vi "Event Builder.vi"() -> ()   [LabVIEW 2021]
uses:
  CamState.ctl
  <userlib>/FTools/JSON Pretty Printer/JSON Pretty Printer.lvlib
  <vilib>/DAQmx/create/channels.llb/DAQmx Create Channel (DO-Digital Output).vi
  <vilib>/DAQmx/write.llb/DAQmx Write (Digital Bool 1Line 1Point).vi
  <vilib>/DAQmx/create/channels.llb/DAQmx Create Channel (DI-Digital Input).vi
  <vilib>/Field R&D Services/LIBSSH2 for LabVIEW/Toolkit/Channel/Channel.lvclass
  <vilib>/DAQmx/write.llb/DAQmx Write (Digital 1D Bool 1Chan 1Samp).vi
  <vilib>/DAQmx/read.llb/DAQmx Read (Digital 1D Bool 1Chan 1Samp).vi
  <vilib>/DAQmx/read.llb/DAQmx Read (Digital Bool 1Line 1Point).vi
  CamConfig.ctl
panel:
  in  "Preview Cam":enum32{"cam0.local", "cam1.local", "cam2.local"}(radio)
  in  "Preview":bool
  out "cam ip":string[](array[string])=["cam0.local", "cam2.local"]
  out "Enum":T1
  in  "Tab Control":enum32{"Log", "Configuration"}(tab)
  in  "Show Latest":bool
  out "text":string
  in  "Camera Configuration":T2
  in  "Save Config":bool
  out "trig latch":tag="Dev1/port2/line1"
  out "state":tag="Dev1/port2/line5, Dev1/port1/line5, Dev1/port1/line0"
  out "trig reset":tag="Dev1/port2/line0"
  out "trig":tag="Dev1/port2/line1"
  out "enable":tag="Dev1/port2/line5, Dev1/port1/line5, Dev1/port1/line0"
  out "state_com":tag="Dev1/port2/line5, Dev1/port1/line5, Dev1/port1/line0"
  out "Trig Enabled":bool caption="Time has Elapsed"
  in  "Timer Reset":bool
  out "Camera Status":u32[](array[colorbox])
  in  "Start Event":bool
  in  "Manual Trigger":bool
  in  "Capture Frane":bool
  in  "Quit":bool
  out "Event":u32
  out "Time Elapsed (s)":dbl format="%.3f"
  out "Run":string
  out "Triggered":bool
  out "Path":string="C:\\Users\\SBC\\Documents\\Camera_Data\\"
  out "config_path":path=path "C:/Users/SBC/Documents/SBC-EventBuilder/camera_config.json"
  # "Cam 0"
  # "Cam 1"
  # "Cam 2"
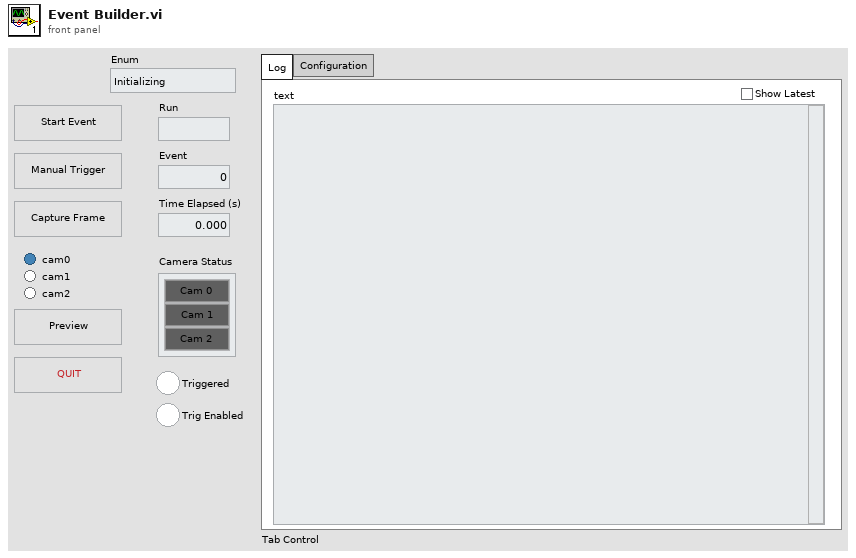
[diagram p1: front panel]
types:
  T1 = typedef "CamState.ctl" = enum16{"Initializing", "Idle", "Starting Event", "Starting RPi", "During Event", "Reset", "Reset RPi", "Preview", "Quit"}
  T2 = typedef "CamConfig.ctl" = cluster{"exposure":u32, "resolution":u32[], "frame_sync":bool, "mode":u32, "buffer_len":u32, "frames_after":u32, "adc_threshold":u32, "pix_threshold":u32, "save_path":string, "config_path":string, "cam_name":string, "image_format":string, "date_format":string, "input_pins":cluster{"state_com":u8, "trig_en":u8, "trig_latch":u8}, "output_pins":cluster{"state":u8, "trig":u8}}
  T3 = enum8{"Enabled", "Disabled", "Disabled and Grayed Out"}
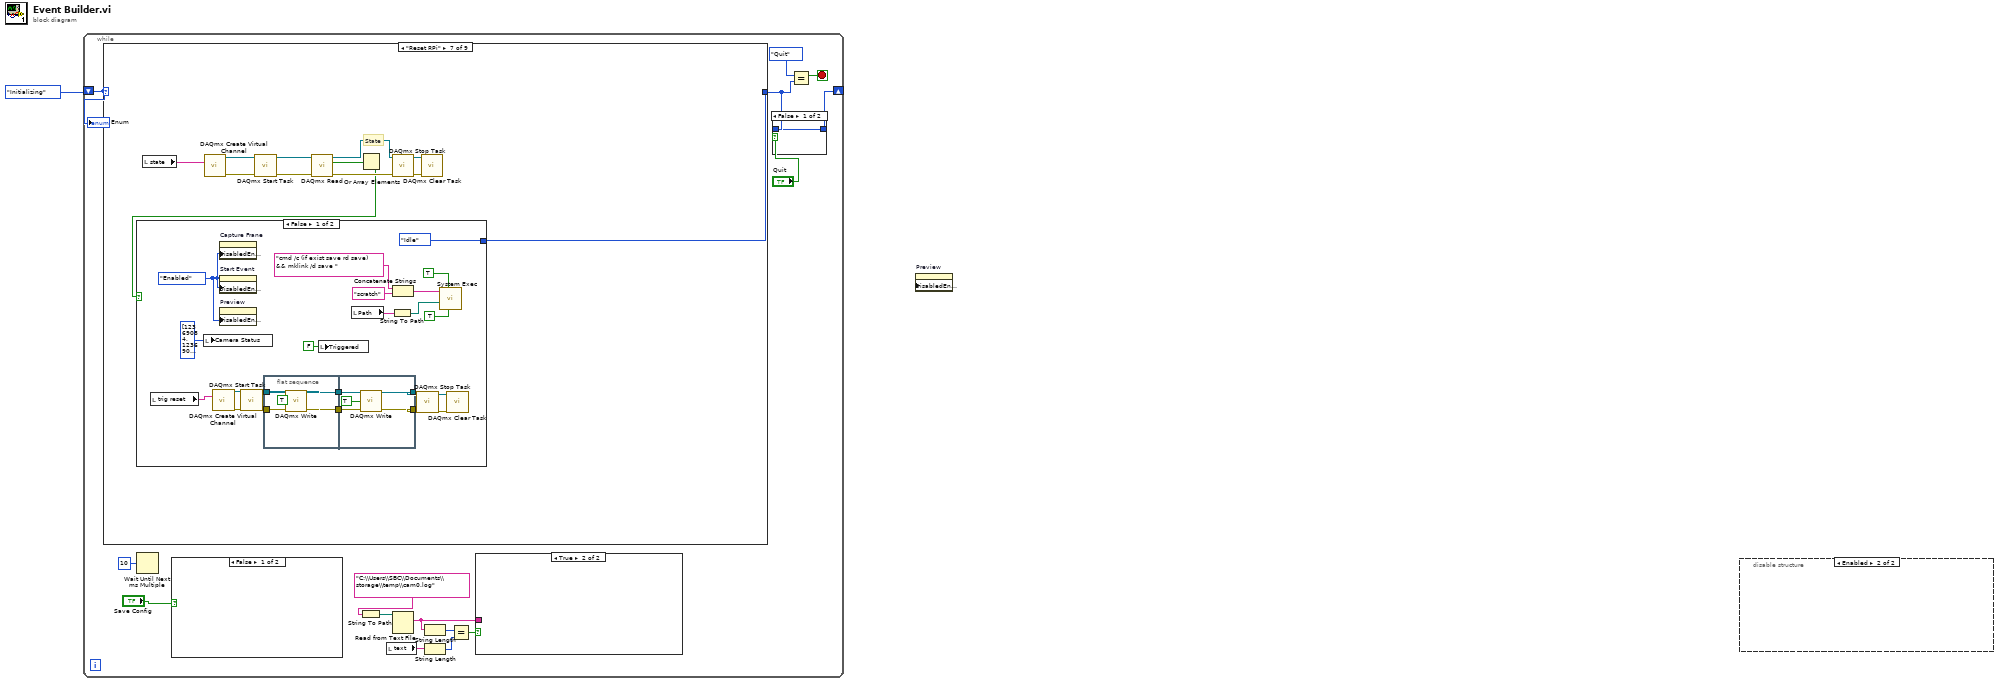
[diagram p0: block diagram]
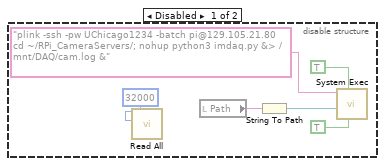
[diagram p2: hidden frame]
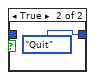
[diagram p3: hidden frame]
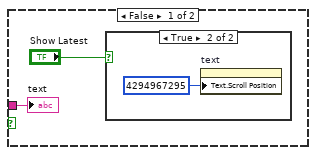
[diagram p4: hidden frame]
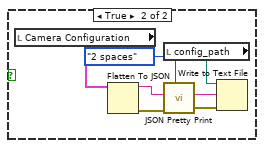
[diagram p6: hidden frame]
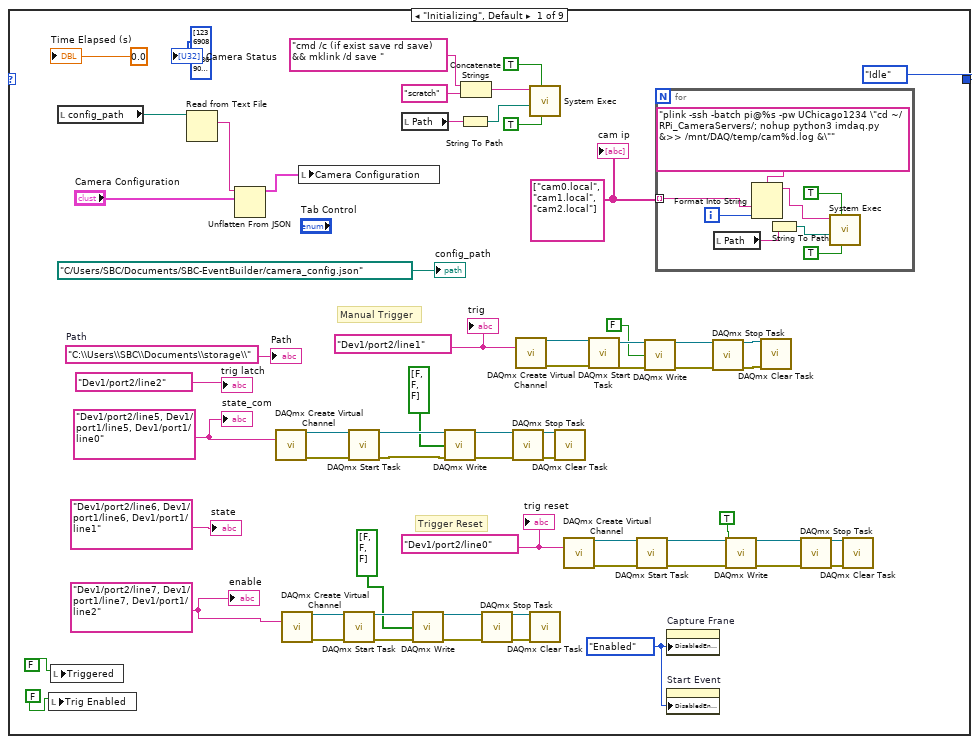
[diagram p7: hidden frame]
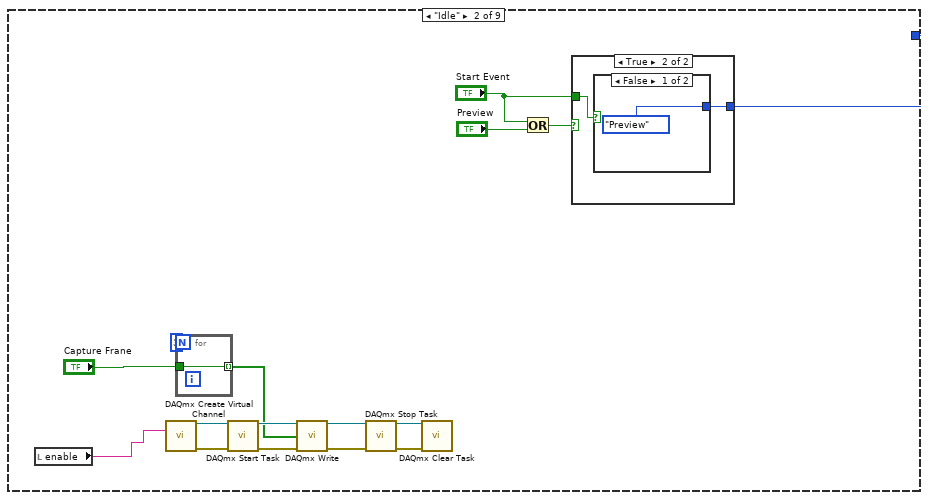
[diagram p8: hidden frame]
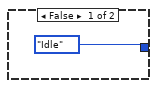
[diagram p9: hidden frame]
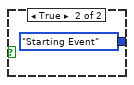
[diagram p10: hidden frame]
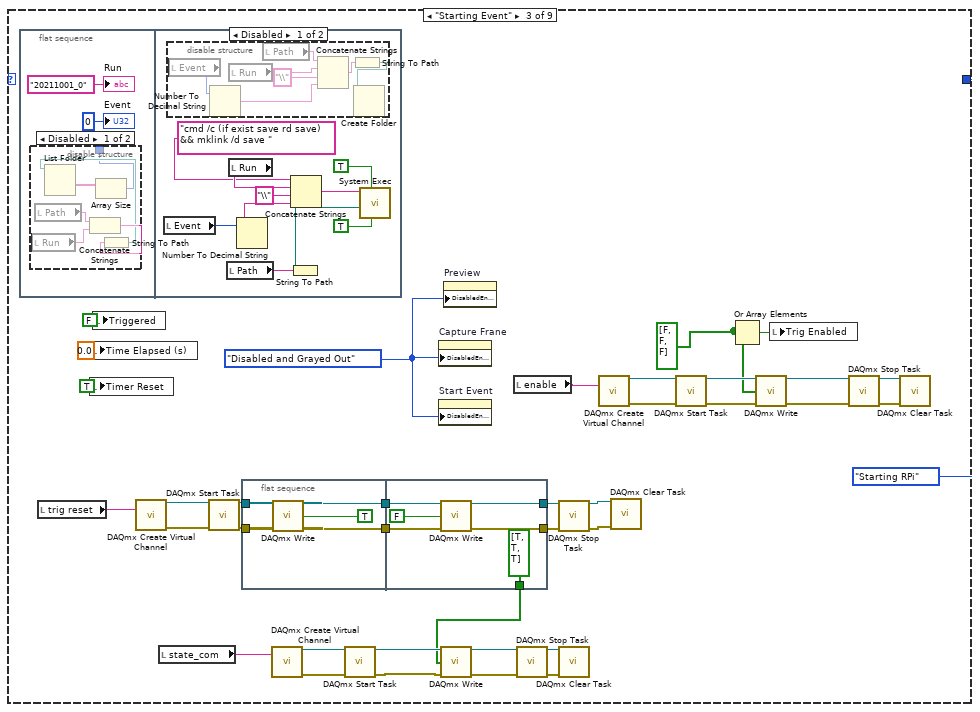
[diagram p11: hidden frame]
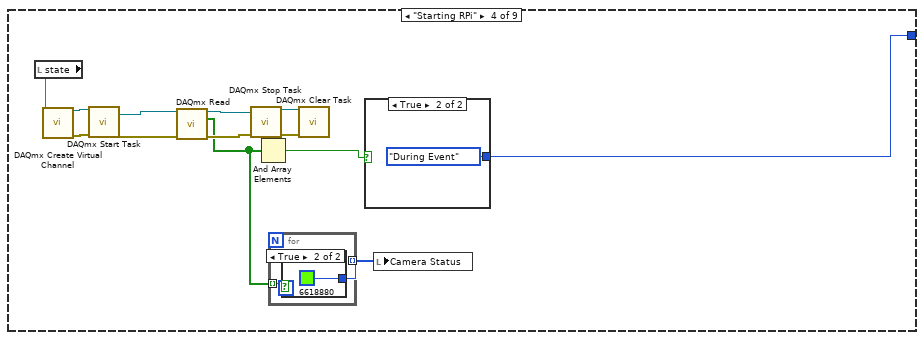
[diagram p14: hidden frame]
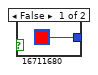
[diagram p15: hidden frame]
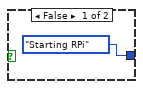
[diagram p16: hidden frame]
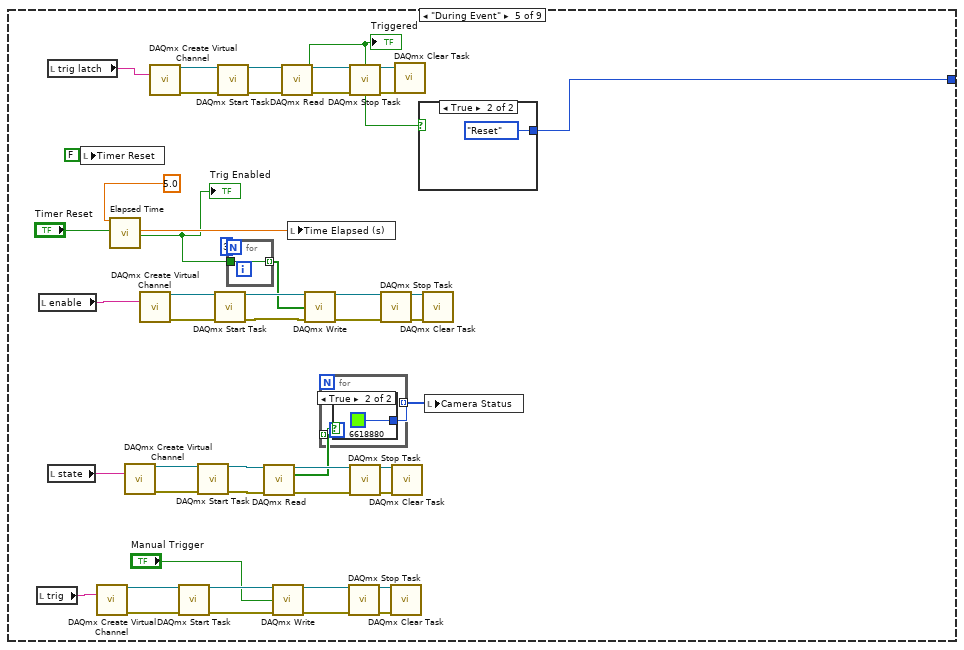
[diagram p17: hidden frame]
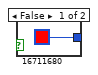
[diagram p18: hidden frame]
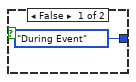
[diagram p19: hidden frame]
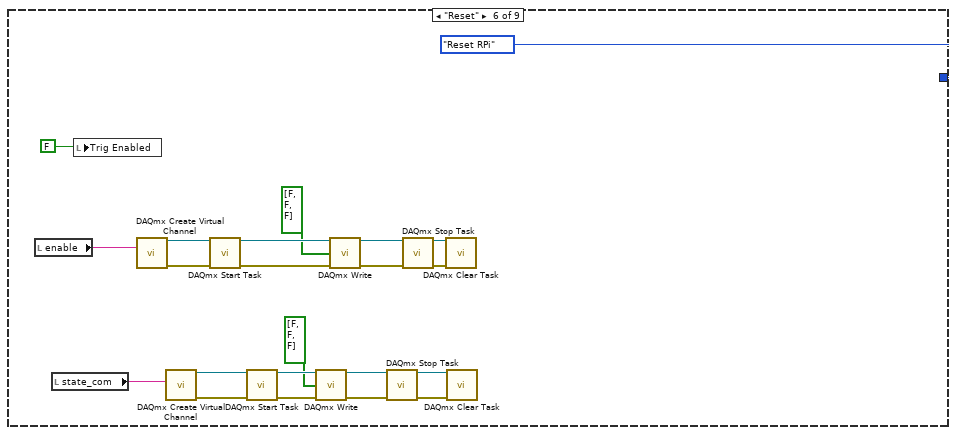
[diagram p20: hidden frame]
diagram:
  n1 = while {
    shift-right: [w5] -> _
    shift-left: CamState."Initializing" -> [w16]
    stop <- w2 stop-if-true
    n2 = case shown="\"Reset RPi\"" w16 {
      tunnel: [CamState."Idle" w114 CamState."Starting RPi" w196 w260 CamState."Reset RPi" w290 CamState."Idle" w365] -> w3
      frame "Initializing", Default {
        w29 = string[] ["cam0.local", "cam1.local", "cam2.local"]
        w32 = tag "Dev1/port2/line7, Dev1/port1/line7, Dev1/port1/line2" ("lines")
        w35 = tag "Dev1/port2/line5, Dev1/port1/line5, Dev1/port1/line0" ("lines")
        w43 = tag "Dev1/port2/line0" ("lines")
        w63 = T3."Enabled" ("Disabled")
        w69 = tag "Dev1/port2/line1" ("lines")
        w62 = "C:\\Users\\SBC\\Documents\\storage\\"  # Path
        # "Trigger Reset"
        # "Manual Trigger"
        n3 = local write "Trig Enabled"(FALSE ("Trig Enabled")) -> ()
        n4 = local write "Triggered"(FALSE ("Triggered")) -> ()
        n5 = local read "config_path"() -> (w86:path)
        n6 = Read from Text File(file (use dialog)=w86) -> (text=w85:string)  [unwired: 3 in, 3 out]
        n7 = Unflatten From JSON(JSON string=w85, type and defaults="Camera Configuration") -> (value=w83:T2)  [unwired: 5 in, 1 out]
        n8 = call-poly <vilib>:"DAQmx Create Virtual Channel.vi"("lines"=w35) -> ("task out"=w53:refnum<k21>, "error out"=w52:errorcluster)  [unwired: 13 in]
        n9 = call-poly <vilib>:"DAQmx Create Virtual Channel.vi"("lines"=w32) -> ("task out"=w79:refnum<k21>, "error out"=w78:errorcluster)  [unwired: 13 in]
        n10 = local write "Camera Configuration"(w83) -> ()
        n11 = call <vilib>:"DAQmx Start Task.vi"("task/channels in"=w79, "error in"=w78) -> ("task out"=w77:refnum<k21>, "error out"=w76:errorcluster)  [unwired: 12 in]
        n12 = call <vilib>:"DAQmx Start Task.vi"("task/channels in"=w53, "error in"=w52) -> ("task out"=w51:refnum<k21>, "error out"=w50:errorcluster)  [unwired: 12 in]
        n13 = local read "Path"() -> (w60:string)
        n14 = call-poly <vilib>:"DAQmx Write.vi"("task/channels in"=w77, "data"=bool[] [FALSE, FALSE, FALSE], "error in"=w76) -> ("task out"=w75:refnum<k21>, "error out"=w74:errorcluster)  [unwired: 10 in, 1 out]
        n15 = call-poly <vilib>:"DAQmx Write.vi"("task/channels in"=w51, "data"=bool[] [FALSE, FALSE, FALSE], "error in"=w50) -> ("task out"=w49:refnum<k21>, "error out"=w48:errorcluster)  [unwired: 10 in, 1 out]
        n16 = String To Path(string=w60) -> (path=w59:path)
        n17 = Concatenate Strings("cmd /c (if exist save rd save) && mklink /d save " ("string"), "scratch" ("string")) -> (w61:string)
        n18 = call <vilib>:"DAQmx Stop Task.vi"("task/channels in"=w75, "error in"=w74) -> ("task out"=w81:refnum<k21>, "error out"=w80:errorcluster)  [unwired: 12 in]
        n19 = call <vilib>:"DAQmx Stop Task.vi"("task/channels in"=w49, "error in"=w48) -> ("task out"=w55:refnum<k21>, "error out"=w54:errorcluster)  [unwired: 12 in]
        n20 = call-poly <vilib>:"DAQmx Create Virtual Channel.vi"("lines"=w69) -> ("task out"=w71:refnum<k21>, "error out"=w70:errorcluster)  [unwired: 13 in]
        n21 = call <vilib>:"System Exec.vi"("run minimized? (F)"=TRUE, "wait until completion? (T)"=TRUE, "working directory"=w59, "command line"=w61) -> ()  [unwired: 4 in, 4 out]
        n22 = call <vilib>:"DAQmx Clear Task.vi"("task in"=w81, "error in"=w80) -> ()  [unwired: 13 in, 1 out]
        n23 = call <vilib>:"DAQmx Clear Task.vi"("task in"=w55, "error in"=w54) -> ()  [unwired: 13 in, 1 out]
        n24 = call-poly <vilib>:"DAQmx Create Virtual Channel.vi"("lines"=w43) -> ("task out"=w45:refnum<k21>, "error out"=w44:errorcluster)  [unwired: 13 in]
        n25 = call <vilib>:"DAQmx Start Task.vi"("task/channels in"=w71, "error in"=w70) -> ("task out"=w68:refnum<k21>, "error out"=w67:errorcluster)  [unwired: 12 in]
        n26 = call <vilib>:"DAQmx Start Task.vi"("task/channels in"=w45, "error in"=w44) -> ("task out"=w41:refnum<k21>, "error out"=w40:errorcluster)  [unwired: 12 in]
        n27 = call-poly <vilib>:"DAQmx Write.vi"("task/channels in"=w68, "data"=FALSE, "error in"=w67) -> ("task out"=w65:refnum<k21>, "error out"=w66:errorcluster)  [unwired: 10 in, 1 out]
        n28 = for {
          tunnel: w29 -> [w92] mode=indexing
          i -> [w91]
          n29 = local read "Path"() -> (w98:string)
          n30 = Format Into String(format string="plink -ssh -batch pi@%s -pw UChicago1234 \"cd ~/RPi_CameraServers/; nohup python3 imdaq.py &>> /mnt/DAQ/temp/cam%d.log &\"" ("string"), w92, w91) -> (resulting string=w93:string)  [unwired: 2 in, 1 out]
          n31 = String To Path(string=w98) -> (path=w97:path)
          n32 = call <vilib>:"System Exec.vi"("run minimized? (F)"=TRUE, "wait until completion? (T)"=TRUE, "working directory"=w97, "command line"=w93) -> ()  [unwired: 4 in, 4 out]
        }
        n33 = property on="Capture Frane" class="Bool"("DisabledEnum"=w63) -> ()  [unwired: 2 in, 2 out]
        n34 = property on="Start Event" class="Bool"("DisabledEnum"=w63) -> ()  [unwired: 2 in, 2 out]
        n35 = call <vilib>:"DAQmx Stop Task.vi"("task/channels in"=w65, "error in"=w66) -> ("task out"=w73:refnum<k21>, "error out"=w72:errorcluster)  [unwired: 12 in]
        n36 = call-poly <vilib>:"DAQmx Write.vi"("task/channels in"=w41, "data"=TRUE, "error in"=w40) -> ("task out"=w39:refnum<k21>, "error out"=w38:errorcluster)  [unwired: 10 in, 1 out]
        n37 = call <vilib>:"DAQmx Clear Task.vi"("task in"=w73, "error in"=w72) -> ()  [unwired: 13 in, 1 out]
        n38 = call <vilib>:"DAQmx Stop Task.vi"("task/channels in"=w39, "error in"=w38) -> ("task out"=w47:refnum<k21>, "error out"=w46:errorcluster)  [unwired: 12 in]
        n39 = call <vilib>:"DAQmx Clear Task.vi"("task in"=w47, "error in"=w46) -> ()  [unwired: 13 in, 1 out]
        "Time Elapsed (s)" <- 0.0 ("Time Elapsed")
        "Camera Status" <- u32[] [12369084, 12369084, 12369084] ("Array")
        "config_path" <- path "C:/Users/SBC/Documents/SBC-EventBuilder/camera_config.json" ("file (use dialog)")
        "Path" <- w62
        "state_com" <- w35
        "enable" <- w32
        "trig" <- w69
        "trig reset" <- w43
        "state" <- tag "Dev1/port2/line6, Dev1/port1/line6, Dev1/port1/line1" ("lines")
        "trig latch" <- tag "Dev1/port2/line2" ("lines")
        "cam ip" <- w29
      }
      frame "Idle" {
        n40 = local read "enable"() -> (w113:tag)
        n41 = call-poly <vilib>:"DAQmx Create Virtual Channel.vi"("lines"=w113) -> ("task out"=w110:refnum<k21>, "error out"=w109:errorcluster)  [unwired: 13 in]
        n42 = for {
          N: 3 -> [_]
          tunnel: [w115] -> w102 mode=indexing
          tunnel: "Capture Frane" -> [w115]
        }
        n43 = call <vilib>:"DAQmx Start Task.vi"("task/channels in"=w110, "error in"=w109) -> ("task out"=w108:refnum<k21>, "error out"=w107:errorcluster)  [unwired: 12 in]
        n44 = call-poly <vilib>:"DAQmx Write.vi"("task/channels in"=w108, "data"=w102, "error in"=w107) -> ("task out"=w106:refnum<k21>, "error out"=w105:errorcluster)  [unwired: 10 in, 1 out]
        n45 = call <vilib>:"DAQmx Stop Task.vi"("task/channels in"=w106, "error in"=w105) -> ("task out"=w112:refnum<k21>, "error out"=w111:errorcluster)  [unwired: 12 in]
        n46 = call <vilib>:"DAQmx Clear Task.vi"("task in"=w112, "error in"=w111) -> ()  [unwired: 13 in, 1 out]
        n47 = Or(x="Start Event", y="Preview") -> (x .or. y?=w100:bool)
        n48 = case shown="True" w100 {
          tunnel: [CamState."Idle" w118] -> w114
          tunnel: "Start Event" -> [_ w117]
          frame False {
          }
          frame True {
            n49 = case shown="False" w117 {
              tunnel: [CamState."Preview" CamState."Starting Event"] -> w118
              frame False {
              }
              frame True {
              }
            }
          }
        }
      }
      frame "Starting Event" {
        w134 = bool[] [FALSE, FALSE, FALSE] ("data")
        w121 = T3."Disabled and Grayed Out" ("Disabled")
        n50 = flat-sequence {
          frame #0 {
            n51 = disable-structure shown="Disabled" {
              disable-tunnel: [w171 _] -> _
              frame Disabled {
                n52 = local read "Run"() -> (w175:string)
                n53 = local read "Path"() -> (w174:string)
                n54 = Concatenate Strings(w174, w175) -> (w173:string)
                n55 = String To Path(string=w173) -> (path=w172:path)
                n56 = List Folder(path=w172) -> (folder names=w176:string[])  [unwired: 3 in, 3 out]
                n57 = Array Size(array=w176) -> (size(s)=w171:i32)
              }
              frame Enabled {
              }
            }
            "Event" <- u32 0 ("Event")
            "Run" <- "20211001_0" ("Run")
          }
          frame #1 {
            n58 = local read "Event"() -> (w181:u32)
            n59 = disable-structure shown="Disabled" {
              frame Disabled {
                n60 = local read "Event"() -> (w188:u32)
                n61 = Number To Decimal String(number=w188) -> (decimal integer string=w187:string)  [unwired: 1 in]
                n62 = local read "Run"() -> (w192:string)
                n63 = local read "Path"() -> (w193:string)
                n64 = Concatenate Strings(w193, w192, "\\" ("string"), w187) -> (w191:string)
                n65 = String To Path(string=w191) -> (path=w190:path)
                n66 = Create Folder(path (use dialog)=w190) -> ()  [unwired: 2 in, 3 out]
              }
              frame Enabled {
              }
            }
            n67 = local read "Path"() -> (w184:string)
            n68 = local read "Run"() -> (w182:string)
            n69 = Number To Decimal String(number=w181) -> (decimal integer string=w180:string)  [unwired: 1 in]
            n70 = String To Path(string=w184) -> (path=w183:path)
            n71 = Concatenate Strings("cmd /c (if exist save rd save) && mklink /d save " ("string"), w182, "\\" ("string"), w180) -> (w186:string)
            n72 = call <vilib>:"System Exec.vi"("run minimized? (F)"=TRUE, "wait until completion? (T)"=TRUE, "working directory"=w183, "command line"=w186) -> ()  [unwired: 4 in, 4 out]
          }
        }
        n73 = local read "trig reset"() -> (w133:tag)
        n74 = local write "Time Elapsed (s)"(0.0 ("Time Elapsed (s)")) -> ()
        n75 = local write "Timer Reset"(TRUE ("Timer Reset")) -> ()
        n76 = local write "Triggered"(FALSE ("Triggered")) -> ()
        n77 = call-poly <vilib>:"DAQmx Create Virtual Channel.vi"("lines"=w133) -> ("task out"=w153:refnum<k21>, "error out"=w152:errorcluster)  [unwired: 13 in]
        n78 = local read "state_com"() -> (w123:tag)
        n79 = call <vilib>:"DAQmx Start Task.vi"("task/channels in"=w153, "error in"=w152) -> ("task out"=w151:refnum<k21>, "error out"=w150:errorcluster)  [unwired: 12 in]
        n80 = flat-sequence {
          tunnel: w151 -> [w162]
          tunnel: w150 -> [w161]
          tunnel: [w159] -> w147
          tunnel: [w158] -> w146
          tunnel: [w168] -> w149
          tunnel: [w167] -> w148
          tunnel: w147 -> [w165]
          tunnel: w146 -> [w164]
          tunnel: [bool[] [TRUE, TRUE, TRUE] ("data")] -> w122
          frame #0 {
            n81 = call-poly <vilib>:"DAQmx Write.vi"("task/channels in"=w162, "data"=TRUE, "error in"=w161) -> ("task out"=w158:refnum<k21>, "error out"=w159:errorcluster)  [unwired: 10 in, 1 out]
          }
          frame #1 {
            n82 = call-poly <vilib>:"DAQmx Write.vi"("task/channels in"=w164, "data"=FALSE, "error in"=w165) -> ("task out"=w168:refnum<k21>, "error out"=w167:errorcluster)  [unwired: 10 in, 1 out]
          }
        }
        n83 = call-poly <vilib>:"DAQmx Create Virtual Channel.vi"("lines"=w123) -> ("task out"=w129:refnum<k21>, "error out"=w128:errorcluster)  [unwired: 13 in]
        n84 = call <vilib>:"DAQmx Start Task.vi"("task/channels in"=w129, "error in"=w128) -> ("task out"=w127:refnum<k21>, "error out"=w126:errorcluster)  [unwired: 12 in]
        n85 = property on="Capture Frane" class="Bool"("DisabledEnum"=w121) -> ()  [unwired: 2 in, 2 out]
        n86 = property on="Start Event" class="Bool"("DisabledEnum"=w121) -> ()  [unwired: 2 in, 2 out]
        n87 = call-poly <vilib>:"DAQmx Write.vi"("task/channels in"=w127, "data"=w122, "error in"=w126) -> ("task out"=w125:refnum<k21>, "error out"=w124:errorcluster)  [unwired: 10 in, 1 out]
        n88 = property on="Preview" class="Bool"("DisabledEnum"=w121) -> ()  [unwired: 2 in, 2 out]
        n89 = local read "enable"() -> (w136:tag)
        n90 = call <vilib>:"DAQmx Stop Task.vi"("task/channels in"=w125, "error in"=w124) -> ("task out"=w131:refnum<k21>, "error out"=w130:errorcluster)  [unwired: 12 in]
        n91 = call <vilib>:"DAQmx Stop Task.vi"("task/channels in"=w149, "error in"=w148) -> ("task out"=w155:refnum<k21>, "error out"=w154:errorcluster)  [unwired: 12 in]
        n92 = call <vilib>:"DAQmx Clear Task.vi"("task in"=w131, "error in"=w130) -> ()  [unwired: 13 in, 1 out]
        n93 = call-poly <vilib>:"DAQmx Create Virtual Channel.vi"("lines"=w136) -> ("task out"=w143:refnum<k21>, "error out"=w142:errorcluster)  [unwired: 13 in]
        n94 = call <vilib>:"DAQmx Clear Task.vi"("task in"=w155, "error in"=w154) -> ()  [unwired: 13 in, 1 out]
        n95 = call <vilib>:"DAQmx Start Task.vi"("task/channels in"=w143, "error in"=w142) -> ("task out"=w141:refnum<k21>, "error out"=w140:errorcluster)  [unwired: 12 in]
        n96 = Or Array Elements(Boolean array=w134) -> (logical OR=w135:bool)
        n97 = call-poly <vilib>:"DAQmx Write.vi"("task/channels in"=w141, "data"=w134, "error in"=w140) -> ("task out"=w139:refnum<k21>, "error out"=w138:errorcluster)  [unwired: 10 in, 1 out]
        n98 = local write "Trig Enabled"(w135) -> ()
        n99 = call <vilib>:"DAQmx Stop Task.vi"("task/channels in"=w139, "error in"=w138) -> ("task out"=w145:refnum<k21>, "error out"=w144:errorcluster)  [unwired: 12 in]
        n100 = call <vilib>:"DAQmx Clear Task.vi"("task in"=w145, "error in"=w144) -> ()  [unwired: 13 in, 1 out]
      }
      frame "Starting RPi" {
        n101 = local read "state"() -> (w200:tag)
        n102 = call-poly <vilib>:"DAQmx Create Virtual Channel.vi"("lines"=w200) -> ("task out"=w199:refnum<k21>, "error out"=w204:errorcluster)  [unwired: 13 in]
        n103 = call <vilib>:"DAQmx Start Task.vi"("task/channels in"=w199, "error in"=w204) -> ("task out"=w198:refnum<k21>, "error out"=w203:errorcluster)  [unwired: 12 in]
        n104 = call-poly <vilib>:"DAQmx Read.vi"("task/channels in"=w198, "error in"=w203) -> ("task out"=w202:refnum<k21>, "data"=w194:bool[], "error out"=w201:errorcluster)  [unwired: 11 in]
        n105 = call <vilib>:"DAQmx Stop Task.vi"("task/channels in"=w202, "error in"=w201) -> ("task out"=w206:refnum<k21>, "error out"=w205:errorcluster)  [unwired: 12 in]
        n106 = And Array Elements(Boolean array=w194) -> (logical AND=w197:bool)
        n107 = for {
          tunnel: [w208] -> w195 mode=indexing
          tunnel: w194 -> [w207] mode=indexing
          n108 = case shown="True" w207 {
            tunnel: [u32 16711680 ("Camera Alive") u32 6618880 ("Camera Alive")] -> w208
            frame False {
            }
            frame True {
            }
          }
        }
        n109 = call <vilib>:"DAQmx Clear Task.vi"("task in"=w206, "error in"=w205) -> ()  [unwired: 13 in, 1 out]
        n110 = case shown="True" w197 {
          tunnel: [CamState."Starting RPi" CamState."During Event"] -> w196
          frame False {
          }
          frame True {
          }
        }
        n111 = local write "Camera Status"(w195) -> ()
      }
      frame "During Event" {
        n112 = local read "trig"() -> (w217:tag)
        n113 = local read "enable"() -> (w220:tag)
        n114 = local read "trig latch"() -> (w218:tag)
        n115 = local read "state"() -> (w219:tag)
        n116 = local write "Timer Reset"(FALSE) -> ()
        n117 = call-poly <vilib>:"DAQmx Create Virtual Channel.vi"("lines"=w217) -> ("task out"=w247:refnum<k21>, "error out"=w246:errorcluster)  [unwired: 13 in]
        n118 = call "Elapsed Time"("Time Target (s)"=5.0, "Reset"="Timer Reset") -> ("Elapsed Time (s)"=w259:dbl, "Time has Elapsed"=w215:bool)  [unwired: 10 in, 6 out]
        "Trig Enabled" <- w215
        n119 = call-poly <vilib>:"DAQmx Create Virtual Channel.vi"("lines"=w219) -> ("task out"=w236:refnum<k21>, "error out"=w237:errorcluster)  [unwired: 13 in]
        n120 = call-poly <vilib>:"DAQmx Create Virtual Channel.vi"("lines"=w220) -> ("task out"=w256:refnum<k21>, "error out"=w255:errorcluster)  [unwired: 13 in]
        n121 = call-poly <vilib>:"DAQmx Create Virtual Channel.vi"("lines"=w218) -> ("task out"=w230:refnum<k21>, "error out"=w231:errorcluster)  [unwired: 13 in]
        n122 = call <vilib>:"DAQmx Start Task.vi"("task/channels in"=w247, "error in"=w246) -> ("task out"=w245:refnum<k21>, "error out"=w244:errorcluster)  [unwired: 12 in]
        n123 = call <vilib>:"DAQmx Start Task.vi"("task/channels in"=w236, "error in"=w237) -> ("task out"=w235:refnum<k21>, "error out"=w234:errorcluster)  [unwired: 12 in]
        n124 = call <vilib>:"DAQmx Start Task.vi"("task/channels in"=w256, "error in"=w255) -> ("task out"=w254:refnum<k21>, "error out"=w253:errorcluster)  [unwired: 12 in]
        n125 = call <vilib>:"DAQmx Start Task.vi"("task/channels in"=w230, "error in"=w231) -> ("task out"=w229:refnum<k21>, "error out"=w228:errorcluster)  [unwired: 12 in]
        n126 = for {
          N: 3 -> [_]
          tunnel: w215 -> [w265]
          tunnel: [w265] -> w214 mode=indexing
        }
        n127 = call-poly <vilib>:"DAQmx Read.vi"("task/channels in"=w235, "error in"=w234) -> ("task out"=w233:refnum<k21>, "data"=w216:bool[], "error out"=w232:errorcluster)  [unwired: 11 in]
        n128 = call-poly <vilib>:"DAQmx Write.vi"("task/channels in"=w245, "data"="Manual Trigger", "error in"=w244) -> ("task out"=w241:refnum<k21>, "error out"=w243:errorcluster)  [unwired: 10 in, 1 out]
        n129 = call-poly <vilib>:"DAQmx Read.vi"("task/channels in"=w229, "error in"=w228) -> ("task out"=w227:refnum<k21>, "data"=w225:bool, "error out"=w226:errorcluster)  [unwired: 11 in]
        "Triggered" <- w225
        n130 = local write "Time Elapsed (s)"(w259) -> ()
        n131 = call-poly <vilib>:"DAQmx Write.vi"("task/channels in"=w254, "data"=w214, "error in"=w253) -> ("task out"=w252:refnum<k21>, "error out"=w251:errorcluster)  [unwired: 10 in, 1 out]
        n132 = for {
          tunnel: [w262] -> w250 mode=indexing
          tunnel: w216 -> [w261] mode=indexing
          n133 = case shown="True" w261 {
            tunnel: [u32 16711680 ("Camera Alive") u32 6618880 ("Camera Alive")] -> w262
            frame False {
            }
            frame True {
            }
          }
        }
        n134 = call <vilib>:"DAQmx Stop Task.vi"("task/channels in"=w241, "error in"=w243) -> ("task out"=w249:refnum<k21>, "error out"=w248:errorcluster)  [unwired: 12 in]
        n135 = call <vilib>:"DAQmx Stop Task.vi"("task/channels in"=w227, "error in"=w226) -> ("task out"=w224:refnum<k21>, "error out"=w223:errorcluster)  [unwired: 12 in]
        n136 = call <vilib>:"DAQmx Stop Task.vi"("task/channels in"=w233, "error in"=w232) -> ("task out"=w222:refnum<k21>, "error out"=w221:errorcluster)  [unwired: 12 in]
        n137 = call <vilib>:"DAQmx Stop Task.vi"("task/channels in"=w252, "error in"=w251) -> ("task out"=w258:refnum<k21>, "error out"=w257:errorcluster)  [unwired: 12 in]
        n138 = call <vilib>:"DAQmx Clear Task.vi"("task in"=w249, "error in"=w248) -> ()  [unwired: 13 in, 1 out]
        n139 = call <vilib>:"DAQmx Clear Task.vi"("task in"=w222, "error in"=w221) -> ()  [unwired: 13 in, 1 out]
        n140 = call <vilib>:"DAQmx Clear Task.vi"("task in"=w224, "error in"=w223) -> ()  [unwired: 13 in, 1 out]
        n141 = case shown="True" w225 {
          tunnel: [CamState."During Event" CamState."Reset"] -> w260
          frame False {
          }
          frame True {
          }
        }
        n142 = call <vilib>:"DAQmx Clear Task.vi"("task in"=w258, "error in"=w257) -> ()  [unwired: 13 in, 1 out]
        n143 = local write "Camera Status"(w250) -> ()
      }
      frame "Reset" {
        n144 = local read "enable"() -> (w271:tag)
        n145 = local read "state_com"() -> (w270:tag)
        n146 = local write "Trig Enabled"(FALSE ("Trig Enabled")) -> ()
        n147 = call-poly <vilib>:"DAQmx Create Virtual Channel.vi"("lines"=w271) -> ("task out"=w287:refnum<k21>, "error out"=w286:errorcluster)  [unwired: 13 in]
        n148 = call-poly <vilib>:"DAQmx Create Virtual Channel.vi"("lines"=w270) -> ("task out"=w279:refnum<k21>, "error out"=w278:errorcluster)  [unwired: 13 in]
        n149 = call <vilib>:"DAQmx Start Task.vi"("task/channels in"=w287, "error in"=w286) -> ("task out"=w285:refnum<k21>, "error out"=w284:errorcluster)  [unwired: 12 in]
        n150 = call <vilib>:"DAQmx Start Task.vi"("task/channels in"=w279, "error in"=w278) -> ("task out"=w277:refnum<k21>, "error out"=w276:errorcluster)  [unwired: 12 in]
        n151 = call-poly <vilib>:"DAQmx Write.vi"("task/channels in"=w277, "data"=bool[] [FALSE, FALSE, FALSE], "error in"=w276) -> ("task out"=w275:refnum<k21>, "error out"=w274:errorcluster)  [unwired: 10 in, 1 out]
        n152 = call-poly <vilib>:"DAQmx Write.vi"("task/channels in"=w285, "data"=bool[] [FALSE, FALSE, FALSE], "error in"=w284) -> ("task out"=w283:refnum<k21>, "error out"=w282:errorcluster)  [unwired: 10 in, 1 out]
        n153 = call <vilib>:"DAQmx Stop Task.vi"("task/channels in"=w275, "error in"=w274) -> ("task out"=w281:refnum<k21>, "error out"=w280:errorcluster)  [unwired: 12 in]
        n154 = call <vilib>:"DAQmx Stop Task.vi"("task/channels in"=w283, "error in"=w282) -> ("task out"=w289:refnum<k21>, "error out"=w288:errorcluster)  [unwired: 12 in]
        n155 = call <vilib>:"DAQmx Clear Task.vi"("task in"=w289, "error in"=w288) -> ()  [unwired: 13 in, 1 out]
        n156 = call <vilib>:"DAQmx Clear Task.vi"("task in"=w281, "error in"=w280) -> ()  [unwired: 13 in, 1 out]
      }
      frame "Reset RPi" {
        # "State"
        n157 = local read "state"() -> (w293:tag)
        n158 = call-poly <vilib>:"DAQmx Create Virtual Channel.vi"("lines"=w293) -> ("task out"=w296:refnum<k21>, "error out"=w297:errorcluster)  [unwired: 13 in]
        n159 = call <vilib>:"DAQmx Start Task.vi"("task/channels in"=w296, "error in"=w297) -> ("task out"=w298:refnum<k21>, "error out"=w299:errorcluster)  [unwired: 12 in]
        n160 = call-poly <vilib>:"DAQmx Read.vi"("task/channels in"=w298, "error in"=w299) -> ("task out"=w300:refnum<k21>, "data"=w292:bool[], "error out"=w301:errorcluster)  [unwired: 11 in]
        n161 = Or Array Elements(Boolean array=w292) -> (logical OR=w291:bool)
        n162 = case shown="False" w291 {
          tunnel: [CamState."Idle" CamState."Reset RPi"] -> w290
          frame False {
            w302 = T3."Enabled" ("Disabled")
            n163 = local read "trig reset"() -> (w303:tag)
            n164 = local write "Camera Status"(u32[] [12369084, 12369084, 12369084] ("Array")) -> ()
            n165 = call-poly <vilib>:"DAQmx Create Virtual Channel.vi"("lines"=w303) -> ("task out"=w309:refnum<k21>, "error out"=w308:errorcluster)  [unwired: 13 in]
            n166 = property on="Capture Frane" class="Bool"("DisabledEnum"=w302) -> ()  [unwired: 2 in, 2 out]
            n167 = property on="Start Event" class="Bool"("DisabledEnum"=w302) -> ()  [unwired: 2 in, 2 out]
            n168 = property on="Preview" class="Bool"("DisabledEnum"=w302) -> ()  [unwired: 2 in, 2 out]
            n169 = call <vilib>:"DAQmx Start Task.vi"("task/channels in"=w309, "error in"=w308) -> ("task out"=w307:refnum<k21>, "error out"=w306:errorcluster)  [unwired: 12 in]
            n170 = flat-sequence {
              tunnel: w307 -> [w328]
              tunnel: w306 -> [w327]
              tunnel: [w325] -> w313
              tunnel: [w324] -> w312
              tunnel: [w333] -> w305
              tunnel: [w332] -> w304
              tunnel: w313 -> [w330]
              tunnel: w312 -> [w329]
              frame #0 {
                n171 = call-poly <vilib>:"DAQmx Write.vi"("task/channels in"=w328, "data"=TRUE, "error in"=w327) -> ("task out"=w324:refnum<k21>, "error out"=w325:errorcluster)  [unwired: 10 in, 1 out]
              }
              frame #1 {
                n172 = call-poly <vilib>:"DAQmx Write.vi"("task/channels in"=w329, "data"=TRUE, "error in"=w330) -> ("task out"=w333:refnum<k21>, "error out"=w332:errorcluster)  [unwired: 10 in, 1 out]
              }
            }
            n173 = local write "Triggered"(FALSE ("Triggered")) -> ()
            n174 = local read "Path"() -> (w321:string)
            n175 = String To Path(string=w321) -> (path=w320:path)
            n176 = Concatenate Strings("cmd /c (if exist save rd save) && mklink /d save " ("string"), "scratch" ("string")) -> (w322:string)
            n177 = call <vilib>:"DAQmx Stop Task.vi"("task/channels in"=w305, "error in"=w304) -> ("task out"=w311:refnum<k21>, "error out"=w310:errorcluster)  [unwired: 12 in]
            n178 = call <vilib>:"System Exec.vi"("run minimized? (F)"=TRUE, "wait until completion? (T)"=TRUE, "working directory"=w320, "command line"=w322) -> ()  [unwired: 4 in, 4 out]
            n179 = call <vilib>:"DAQmx Clear Task.vi"("task in"=w311, "error in"=w310) -> ()  [unwired: 13 in, 1 out]
          }
          frame True {
          }
        }
        n180 = call <vilib>:"DAQmx Stop Task.vi"("task/channels in"=w300, "error in"=w301) -> ("task out"=w294:refnum<k21>, "error out"=w295:errorcluster)  [unwired: 12 in]
        n181 = call <vilib>:"DAQmx Clear Task.vi"("task in"=w294, "error in"=w295) -> ()  [unwired: 13 in, 1 out]
      }
      frame "Preview" {
        (unwired) "cmd /c C:\\\\Program^ Files^ ^(x86^)\\\\gstreamer\\\\1.0\\\\mingw_x86_64\\\\bin\\\\gst-launch-1.0 -v tcpclientsrc host=%s port=%d ! decodebin ! autovideosink" ("command line")
        w350 = 5000 ("input 2")
        n182 = local read "Path"() -> (w349:string)
        n183 = Format Into String(format string="plink -ssh -batch pi@%s -pw UChicago1234 \"pkill -f \\\\\\\"imdaq.py\\\\\\\"\"" ("string"), "Preview Cam") -> (resulting string=w347:string)  [unwired: 2 in, 1 out]
        n184 = String To Path(string=w349) -> (path=w348:path)
        n185 = call <vilib>:"System Exec.vi"("run minimized? (F)"=TRUE, "wait until completion? (T)"=TRUE, "working directory"=w348, "command line"=w347) -> ("error out"=w343:errorcluster)  [unwired: 4 in, 3 out]
        n186 = local read "Path"() -> (w361:string)
        n187 = Format Into String(format string="plink -ssh -batch pi@%s -pw UChicago1234 \"~/RPi_CameraServers/MIPI_Camera/RPI/video2stdout | nc -l -p %d\"" ("string"), "Preview Cam", w350) -> (resulting string=w357:string)  [unwired: 2 in, 1 out]
        n188 = String To Path(string=w361) -> (path=w360:path)
        n189 = call <vilib>:"System Exec.vi"("run minimized? (F)"=TRUE, "wait until completion? (T)"=FALSE, "error in (no error)"=w343, "working directory"=w360, "command line"=w357) -> ("error out"=w354:errorcluster)  [unwired: 3 in, 3 out]
        n190 = local read "Path"() -> (w355:string)
        n191 = Format Into String(format string="C:\\\\Program Files (x86)\\\\gstreamer\\\\1.0\\\\mingw_x86_64\\\\bin\\\\gst-launch-1.0 -v tcpclientsrc host=%s port=%d ! decodebin ! autovideosink" ("command line"), "Preview Cam", w350) -> (resulting string=w351:string)  [unwired: 2 in, 1 out]
        n192 = String To Path(string=w355) -> (path=w364:path)
        n193 = call <vilib>:"System Exec.vi"("run minimized? (F)"=TRUE, "wait until completion? (T)"=TRUE, "error in (no error)"=w354, "working directory"=w364, "command line"=w351) -> ()  [unwired: 3 in, 4 out]
        n194 = local read "Path"() -> (w342:string)
        n195 = Format Into String(format string="plink -ssh -batch pi@%s -pw UChicago1234 \"cd ~/RPi_CameraServers/; nohup python3 imdaq.py &>> /mnt/DAQ/temp/cam%d.log &\"" ("string"), "Preview Cam", 0 ("input 2")) -> (resulting string=w340:string)  [unwired: 2 in, 1 out]
        n196 = String To Path(string=w342) -> (path=w341:path)
        n197 = call <vilib>:"System Exec.vi"("run minimized? (F)"=TRUE, "wait until completion? (T)"=TRUE, "working directory"=w341, "command line"=w340) -> ()  [unwired: 4 in, 4 out]
      }
      frame "Quit" {
        n198 = flat-sequence {
          tunnel: [CamState."Quit"] -> w365
          frame #0 {
            w369 = T3."Enabled" ("Disabled")
            n199 = local write "Camera Status"(u32[] [12369084, 12369084, 12369084] ("Array")) -> ()
            n200 = property on="Capture Frane" class="Bool"("DisabledEnum"=w369) -> ()  [unwired: 2 in, 2 out]
            n201 = property on="Start Event" class="Bool"("DisabledEnum"=w369) -> ()  [unwired: 2 in, 2 out]
            n202 = local read "Path"() -> (w375:string)
            n203 = String To Path(string=w375) -> (path=w374:path)
            n204 = Concatenate Strings("cmd /c (if exist save rd save) && mklink /d save " ("string"), "scratch" ("string")) -> (w376:string)
            n205 = local write "Trig Enabled"(FALSE ("Trig Enabled")) -> ()
            n206 = local write "Triggered"(FALSE ("Triggered")) -> ()
            n207 = call <vilib>:"System Exec.vi"("run minimized? (F)"=TRUE, "wait until completion? (T)"=TRUE, "working directory"=w374, "command line"=w376) -> ()  [unwired: 4 in, 4 out]
          }
          frame #1 {
            n208 = local read "cam ip"() -> (w377:string[])
            n209 = for {
              tunnel: w377 -> [w378] mode=indexing
              n210 = local read "Path"() -> (w384:string)
              n211 = Format Into String(format string="plink -ssh -batch pi@%s -pw UChicago1234 \"pkill -f \\\"imdaq.py\\\"\"" ("string"), w378) -> (resulting string=w379:string)  [unwired: 2 in, 1 out]
              n212 = String To Path(string=w384) -> (path=w383:path)
              n213 = call <vilib>:"System Exec.vi"("run minimized? (F)"=TRUE, "wait until completion? (T)"=TRUE, "working directory"=w383, "command line"=w379) -> ()  [unwired: 4 in, 4 out]
            }
          }
          frame #2 {
          }
        }
      }
    }
    n214 = Wait Until Next ms Multiple(millisecond multiple=u32 10) -> ()  [unwired: 1 out]
    n215 = case shown="False" "Save Config" {
      frame False {
      }
      frame True {
        n216 = local read "Camera Configuration"() -> (w28:T2)
        n217 = Flatten To JSON(anything=w28) -> (JSON string=w26:string, 11:w25:errorcluster)  [unwired: 2 in]
        n218 = local read "config_path"() -> (w27:path)
        n219 = call <userlib>:"JSON Pretty Print.vi"("Identation"=enum16{"tab", "2 spaces"}."2 spaces", "error in"=w25, "JSON String"=w26) -> ("error out"=w23:errorcluster, "JSON Pretty Print Format"=w24:string)  [unwired: 7 in]
        n220 = Write to Text File(file (use dialog)=w27, text=w24, error in=w23) -> ()  [unwired: 1 in, 3 out]
      }
    }
    n221 = String To Path(string="C:\\Users\\SBC\\Documents\\storage\\temp\\cam0.log") -> (path=w8:path)
    n222 = local read "text"() -> (w9:string)
    n223 = Read from Text File(file (use dialog)=w8) -> (text=w13:string)  [unwired: 3 in, 3 out]
    n224 = String Length(string=w13) -> (length=w10:i32)
    n225 = String Length(string=w9) -> (length=w11:i32)
    n226 = Equal?(x=w10, y=w11) -> (x = y?=w12:bool)
    n227 = case shown="True" w12 {
      tunnel: w13 -> [w20 _]
      frame False {
        n228 = case shown="True" "Show Latest" {
          frame False {
          }
          frame True {
            n229 = property on="text" class="Str"("Text.Scroll Position"=u32 4294967295) -> ()  [unwired: 2 in, 2 out]
          }
        }
        "text" <- w20
      }
      frame True {
      }
    }
    n230 = case shown="False" "Quit" {
      tunnel: w3 -> [w17 _]
      tunnel: [w17 CamState."Quit"] -> w5
      frame False {
      }
      frame True {
      }
    }
    n231 = Equal?(x=CamState."Quit", y=w3) -> (x = y?=w2:bool)
    "Enum" <- w16
  }
  n232 = property on="Preview" class="Bool" props=["DisabledEnum"]() -> ()  [unwired: 3 in, 2 out]
  n233 = disable-structure shown="Enabled" {
    frame Disabled {
      n234 = call <vilib>:"Read All.vi"("Max Read Size"=u64 32000 ("Max Data Length")) -> ()  [unwired: 7 in, 4 out]
      n235 = local read "Path"() -> (w390:string)
      n236 = String To Path(string=w390) -> (path=w391:path)
      n237 = call <vilib>:"System Exec.vi"("run minimized? (F)"=TRUE, "wait until completion? (T)"=TRUE, "working directory"=w391, "command line"="plink -ssh -pw UChicago1234 -batch pi@129.105.21.80 cd ~/RPi_CameraServers/; nohup python3 imdaq.py &> /mnt/DAQ/cam.log &") -> ()  [unwired: 4 in, 4 out]
    }
    frame Enabled {
    }
  }
